vi "LDA_Data_1D.vi"(9 "LDA Binary data":u16[][](array[numeric])=array4x1695[6780 elements], 11 "LDA numder":enum16{"LDA 1", "LDA 2"}(ring)) -> (1 "Results Values":dbl[](array[numeric]) format="%.2f", 2 "Results titles":string[](array[string]), 6 "Freq":dbl=25.0 format="%.2f")   [LabVIEW 2010]
uses:
  Globals/LDA_meas_global_1.vi
  Globals/LDA_meas_global_2.vi
panel:
  out "No of Invalid bursts":i32
  out "No of good samples":i32=634
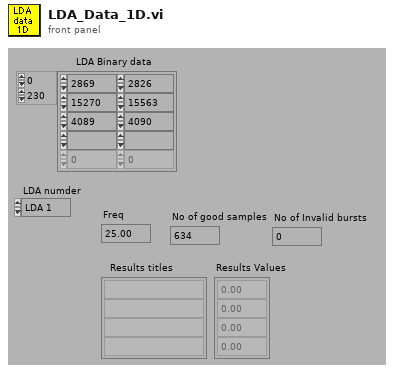
[diagram p1: front panel]
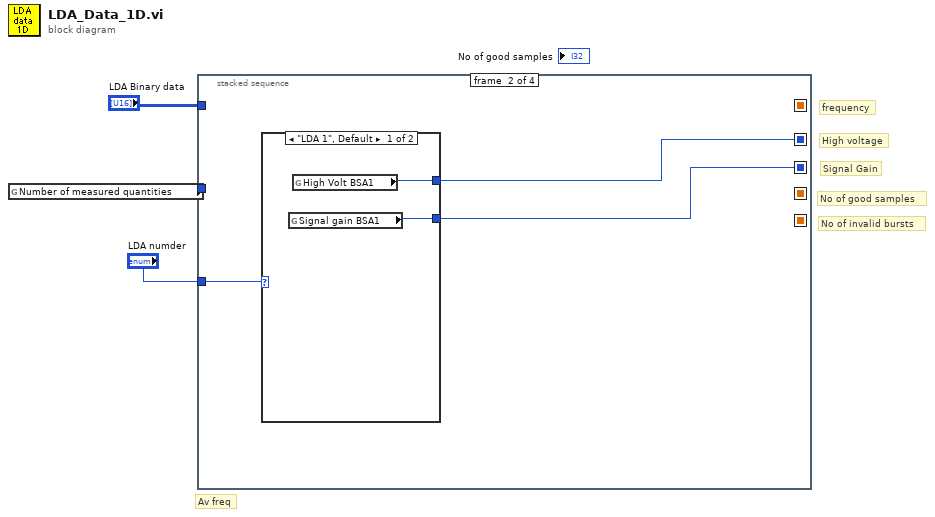
[diagram p0: block diagram]
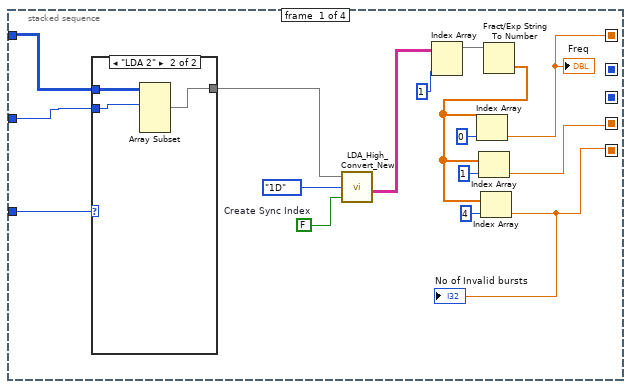
[diagram p2: hidden frame]
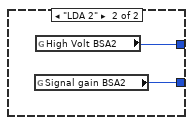
[diagram p4: hidden frame]
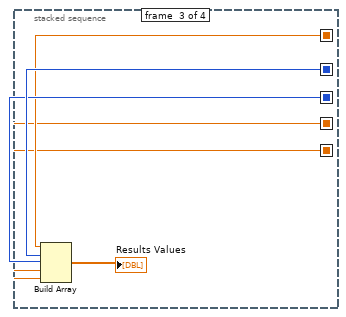
[diagram p5: hidden frame]
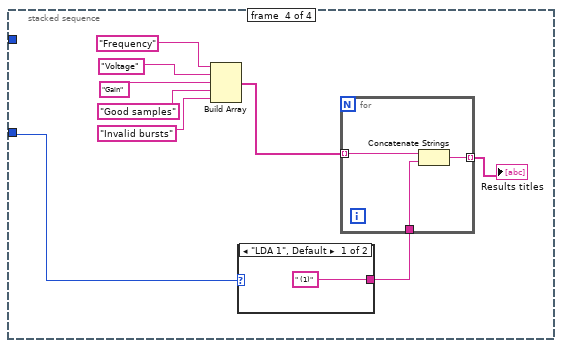
[diagram p6: hidden frame]
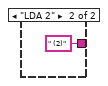
[diagram p7: hidden frame]
diagram:
  # "Signal Gain"
  # "High voltage"
  # "frequency"
  # "No of good samples"
  # "No of invalid bursts"
  # "Av freq"
  n1 = global read "LDA_meas_global_1.vi" "Number of measured quantities"() -> (w3:i32)
  n2 = stacked-sequence {
    seq-local: [w5 _ _ _] -> [_ _ w34 _]
    seq-local: [w6 _ _ _] -> [_ _ w32 _]
    seq-local: [w4 _ _ _] -> [_ _ w31 _]
    seq-local: [_ w25 _ _] -> [_ _ w36 _]
    seq-local: [_ w24 _ _] -> [_ _ w35 _]
    tunnel: "LDA Binary data" -> [w18 _ _ _]
    tunnel: w3 -> [w19 _ _ _]
    tunnel: "LDA numder" -> [w15 w26 _ w40]
    frame #0 {
      w16 = FALSE  # Create Sync Index
      n3 = case shown="\"LDA 2\"" w15 {
        tunnel: [w20 w22] -> w14
        tunnel: w18 -> [w20 w23]
        tunnel: w19 -> [_ w21]
        frame "LDA 1" {
        }
        frame "LDA 2" {
          n4 = Array Subset(array=w23, index (row)=w21) -> (w22:u16[][])  [unwired: 3 in]
        }
      }
      n5 = call "LDA_High_Convert_New.vi"("LDA Binary data"=w14, "dimensions"=enum16{"1D", "2D"}."1D", "Create Sync Index"=w16) -> ("Diagnostic info"=w12:string[][])  [unwired: 3 out]
      n6 = Index Array(array=w12, index (col)=1 ("Index")) -> (element=w11:string[])  [unwired: 1 in]
      n7 = Fract/Exp String To Number(string=w11) -> (number=w7:dbl[])  [unwired: 4 out]
      n8 = Index Array(array=w7, index=0 ("Index")) -> (element=w5:dbl)
      "Freq" <- w5
      n9 = Index Array(array=w7, index=1 ("Index")) -> (element=w6:dbl)
      n10 = Index Array(array=w7, index=4 ("Index")) -> (element=w4:dbl)
      "No of Invalid bursts" <- w4
    }
    frame #1 {
      n11 = case shown="\"LDA 1\", Default" w26 {
        tunnel: [w28 w30] -> w25
        tunnel: [w27 w29] -> w24
        frame "LDA 1", Default {
          n12 = global read "LDA_meas_global_1.vi" "Signal gain BSA1"() -> (w27:i16)
          n13 = global read "LDA_meas_global_1.vi" "High Volt BSA1"() -> (w28:i16)
        }
        frame "LDA 2" {
          n14 = global read "LDA_meas_global_2.vi" "Signal gain BSA2"() -> (w29:i16)
          n15 = global read "LDA_meas_global_2.vi" "High Volt BSA2"() -> (w30:i16)
        }
      }
    }
    frame #2 {
      n16 = Build Array(w34, w36, w35, w32, w31) -> (→"Results Values":dbl[])
    }
    frame #3 {
      n17 = Build Array("Frequency", "Voltage", "Gain", "Good samples", "Invalid bursts") -> (w38:string[])
      n18 = case shown="\"LDA 1\", Default" w40 {
        tunnel: [" (1)" " (2)"] -> w39
        frame "LDA 1", Default {
        }
        frame "LDA 2" {
        }
      }
      n19 = for {
        tunnel: w39 -> [w48]
        tunnel: w38 -> [w47] mode=indexing
        tunnel: [w46] -> w37 mode=indexing
        n20 = Concatenate Strings(w47, w48) -> (w46:string)
      }
      "Results titles" <- w37
    }
  }
